vi "Connect Cable Message.vi"(8 "error in (no error)":errorcluster) -> (0 "error out":errorcluster, 2 "Aborted?":bool)   [LabVIEW 2018]
uses:
  Instrumentation/Door Status Global Variable.vi
panel:
  in  "String":string="Switch the cable in preparation for the Bridgewire and No-Fire Tests"
  in  "Abort":bool
  in  "Continue":bool
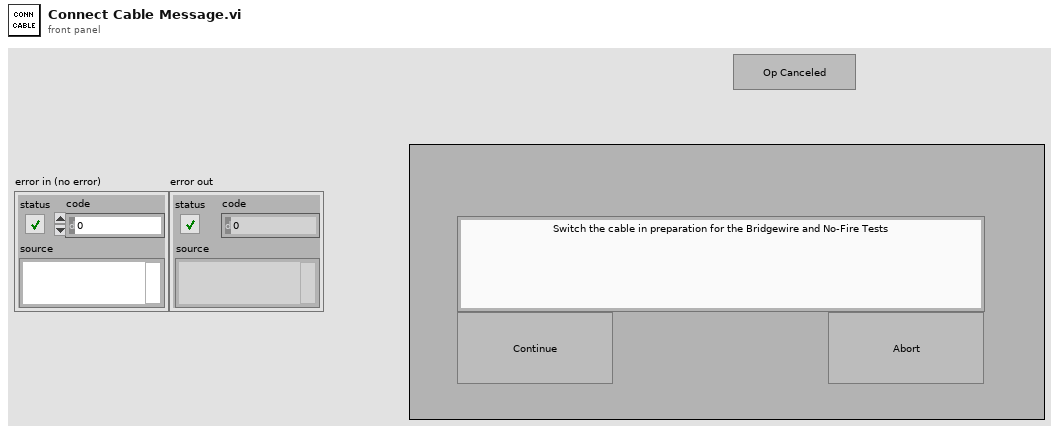
[diagram p1: front panel]
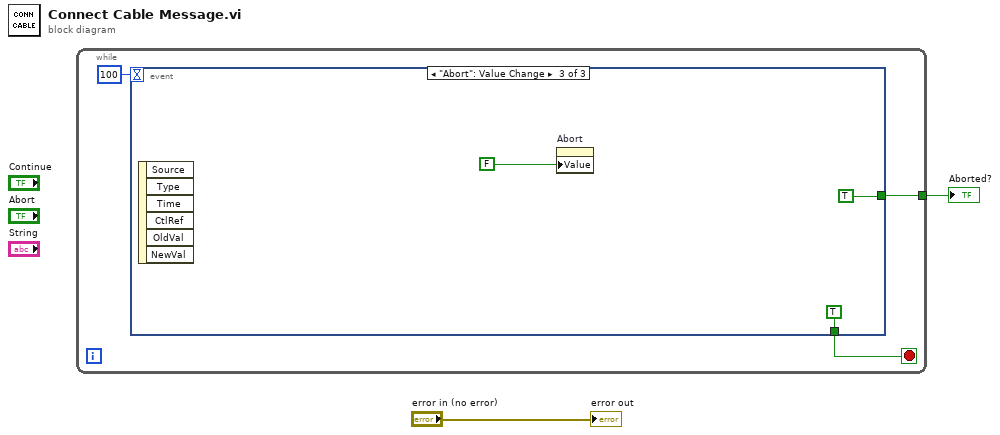
[diagram p0: block diagram]
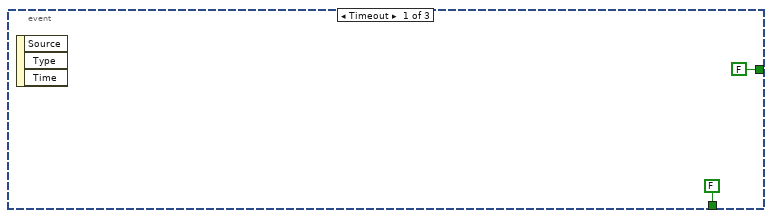
[diagram p2: hidden frame]
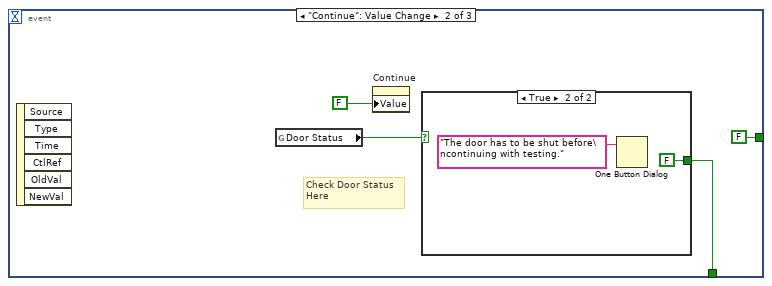
[diagram p3: hidden frame]
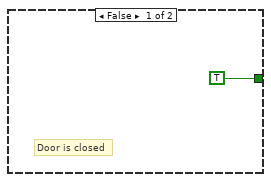
[diagram p4: hidden frame]
diagram:
  n1 = while {
    tunnel: [w4] -> w2
    stop <- w5 stop-if-true
    n2 = event shown="[2] \"Abort\": Value Change" {
      selector: _ -> [_ _ _]
      dyn-events: _ -> [_ _ _]
      timeout: 100 -> [_ _ _]
      tunnel: [FALSE w11 TRUE] -> w5
      tunnel: [FALSE FALSE TRUE] -> w4
      event Timeout {
        n3 = event-data() -> ()  [unwired: 1 in, 3 out]
      }
      event "Continue": Value Change {
        # "Check Door Status\nHere"
        n4 = event-data() -> ()  [unwired: 1 in, 6 out]
        n5 = global read "Door Status Global Variable.vi" "Door Status"() -> (w8:bool)
        n6 = property on="Continue" class="Bool (strict)"("Value"=FALSE ("OK")) -> ()  [unwired: 2 in, 2 out]
        n7 = case shown="True" w8 {
          tunnel: [TRUE FALSE] -> w11
          frame False {
            # "Door is closed"
          }
          frame True {
            n8 = One Button Dialog(message="The door has to be shut before\ncontinuing with testing.") -> ()  [unwired: 1 in, 1 out]
          }
        }
      }
      event "Abort": Value Change {
        n9 = event-data() -> ()  [unwired: 1 in, 6 out]
        n10 = property on="Abort" class="Bool (strict)"("Value"=FALSE ("OK")) -> ()  [unwired: 2 in, 2 out]
      }
    }
  }
  "Aborted?" <- w2
  "error out" <- "error in (no error)"
